vi "Datos imagen.vi"(0 "Refnum in":T1, 1 "Distance (Pixels)":dbl, 2 "Class":string, 3 "empty?":bool) -> (7 "new picture":picture)   [LabVIEW 2021]
uses:
  <vilib>/vision/Image Controls.llb/IMAQ Image.ctl
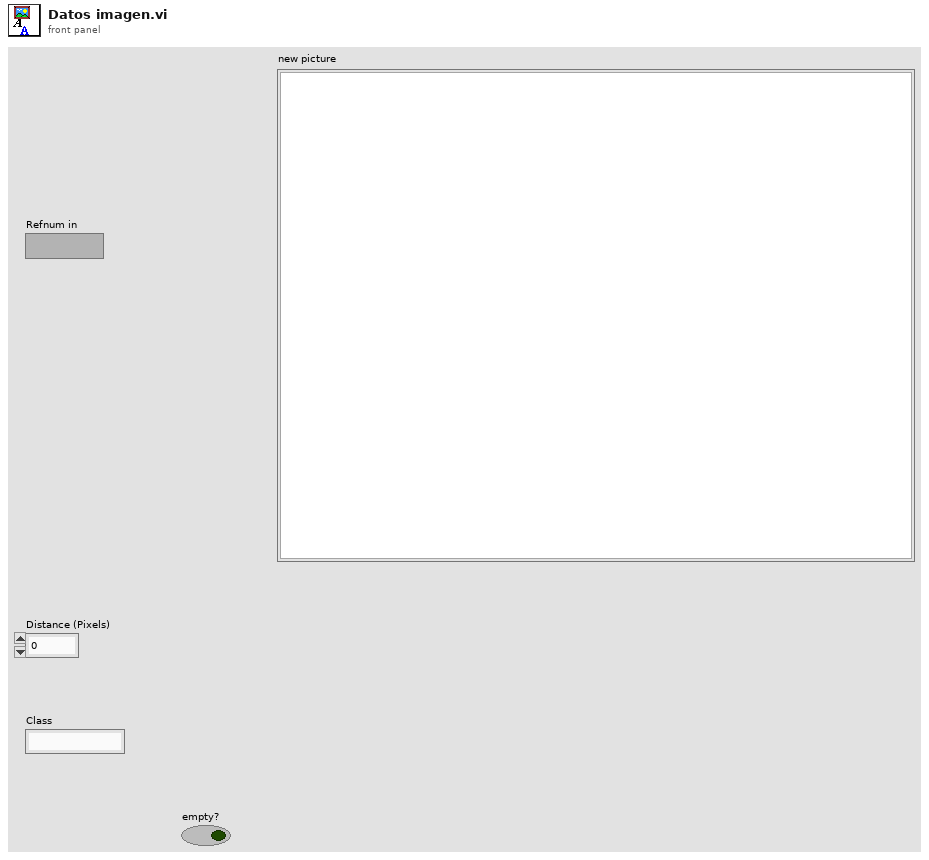
[diagram p1: front panel]
types:
  T1 = typedef "IMAQ Image.ctl" = refnum<image>
  T2 = enum16{"User-specified Font", "Application Font", "System Font", "Dialog Font"}
  T3 = cluster{"Font Name:":string, "Size":i16, "Strikeout?":bool, "Italic?":bool, "Underline?":bool, "Outline?":bool, "Shadow?":bool, "Bold?":bool}
  T4 = cluster{"left":i16, "top":i16, "right":i16, "bottom":i16}
  T5 = typedef "imagedata.ctl" = cluster{"image type":i32, "image depth":i32, "image":u8[], "mask":u8[], "colors":u32[], "Rectangle":cluster{"left":i16, "top":i16, "right":i16, "bottom":i16}}
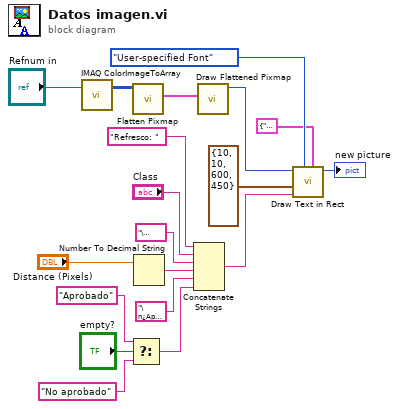
[diagram p0: block diagram]
diagram:
  n1 = call "IMAQ ColorImageToArray"("Image"="Refnum in") -> ("Image Pixels (U32)"=w2:u32[][])  [unwired: 3 in, 2 out]
  n2 = Select(t="Aprobado", s="empty?", f="No aprobado") -> (s? t:f=w15:string)
  n3 = call <vilib>:"Flatten Pixmap.vi"("24-bit pixmap"=w2) -> ("image data"=w3:T5)  [unwired: 10 in]
  n4 = Number To Decimal String(number="Distance (Pixels)") -> (decimal integer string=w14:string)  [unwired: 1 in]
  n5 = Concatenate Strings("Refresco: " ("string"), "Class", "\nDimensión (pixeles): " ("string"), w14, "\n¿Aprobado?: " ("string"), w15) -> (w17:string)
  n6 = call <vilib>:"Draw Flattened Pixmap.vi"("image data"=w3) -> ("new picture"=w4:picture)  [unwired: 8 in]
  n7 = call <vilib>:"Draw Text in Rect.vi"("[user-specified font]"=T3 {"Font Name:"="Arial", "Size"=20, "Strikeout?"=FALSE, "Italic?"=TRUE, "Underline?"=FALSE, "Outline?"=FALSE, "Shadow?"=TRUE, "Bold?"=TRUE}, "desired font(Application)"=T2."User-specified Font", "text"=w17, "rect"=T4 {"left"=10, "top"=10, "right"=600, "bottom"=450}, "picture"=w4) -> ("new picture"=→"new picture":picture)  [unwired: 6 in]
